vi "Close.vi"(8 "error in":errorcluster) -> (0 "error out":errorcluster)   [LabVIEW 2017, in "Game.lvlib" / "GameComms.lvlib"]
uses:
  GameComms.lvlib
  TypeDefs/TCP UDP Ref FGV Commands.ctl
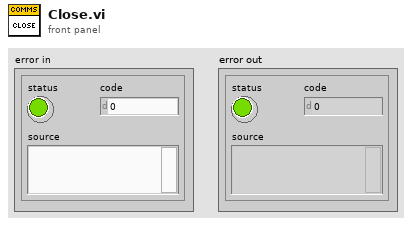
[diagram p1: front panel]
types:
  T1 = typedef "Game.lvlib/GameComms.lvlib/TCP UDP Ref FGV Commands.ctl" = enum16{"Set", "Get"}
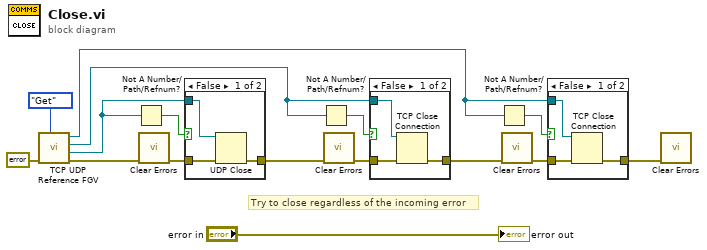
[diagram p0: block diagram]
diagram:
  # "Try to close regardless of the incoming error"
  n1 = call "TCP UDP Reference FGV.vi"("Command"=TCP_UDP_Ref_FGV_Commands."Get", "Error In"=errorcluster {"status"=FALSE, "code"=0, "source"=""}) -> ("Error Out"=w13:errorcluster, "UDP Connection ID"=w10:refnum<k16>, "TCP Connection ID"=w4:refnum<k5>, "TCP Listener ID"=w2:refnum<k5>)  [unwired: 6 in]
  n2 = Not A Number/Path/Refnum?(number/path/refnum=w10) -> (NaN/Path/Refnum?=w11:bool)
  n3 = call <vilib>:"Clear Errors.vi"("error in (no error)"=w13) -> ("error out"=w12:errorcluster)  [unwired: 5 in, 1 out]
  n4 = case shown="False" w11 {
    tunnel: w12 -> [w19 w20]
    tunnel: w10 -> [w18 _]
    tunnel: [w17 w20] -> w5
    frame False {
      n5 = UDP Close(connection ID=w18, 8:w19) -> (error out=w17:errorcluster)  [unwired: 1 out]
    }
    frame True {
    }
  }
  n6 = Not A Number/Path/Refnum?(number/path/refnum=w4) -> (NaN/Path/Refnum?=w9:bool)
  n7 = call <vilib>:"Clear Errors.vi"("error in (no error)"=w5) -> ("error out"=w8:errorcluster)  [unwired: 5 in, 1 out]
  n8 = case shown="False" w9 {
    tunnel: w8 -> [w22 w24]
    tunnel: w4 -> [w21 _]
    tunnel: [w23 w24] -> w3
    frame False {
      n9 = TCP Close Connection(connection ID=w21, error in (no error)=w22) -> (error out=w23:errorcluster)  [unwired: 1 in, 1 out]
    }
    frame True {
    }
  }
  n10 = Not A Number/Path/Refnum?(number/path/refnum=w2) -> (NaN/Path/Refnum?=w6:bool)
  n11 = call <vilib>:"Clear Errors.vi"("error in (no error)"=w3) -> ("error out"=w7:errorcluster)  [unwired: 5 in, 1 out]
  n12 = case shown="False" w6 {
    tunnel: w7 -> [w27 w28]
    tunnel: w2 -> [w25 _]
    tunnel: [w26 w28] -> w1
    frame False {
      n13 = TCP Close Connection(connection ID=w25, error in (no error)=w27) -> (error out=w26:errorcluster)  [unwired: 1 in, 1 out]
    }
    frame True {
    }
  }
  n14 = call <vilib>:"Clear Errors.vi"("error in (no error)"=w1) -> ()  [unwired: 5 in, 2 out]
  "error out" <- "error in"
